vi "数值控件的单位.vi"() -> ()   [LabVIEW 2013]
panel:
  out "面积":dbl[unit]
  in  "宽度":dbl[unit]
  in  "长度":dbl[unit]
  out "秒":dbl[unit]
  in  "时":dbl[unit]
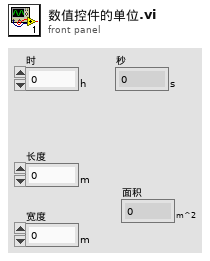
[diagram p1: front panel]
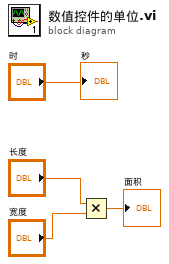
[diagram p0: block diagram]
diagram:
  n1 = Multiply(x="长度", y="宽度") -> (x*y=→"面积":dbl[unit])
  "秒" <- "时"
